vi "Do Action.vi"(8 "error in (no error)":errorcluster, 9 "Display Queue":refnum<queue>, 10 "tlc_User Event Reference.ctl":T1, 11 "Stop in":refnum<class "Stop.lvclass">) -> (0 "error out":errorcluster)   [LabVIEW 2010, in "Stop.lvclass"]
doc: "When the user clicks on the Stop button, this function will be called to halt execution of the cues that have been recorded in the Cue List."
uses:
  Stop.lvclass
  Controls/tlc_User Interface Command.ctl
  Controls/tlc_User Interface Data Type.ctl
  Controls/tlc_User Event Reference.ctl
  Play/Play.lvclass
  Stop.lvclass/Stop.ctl
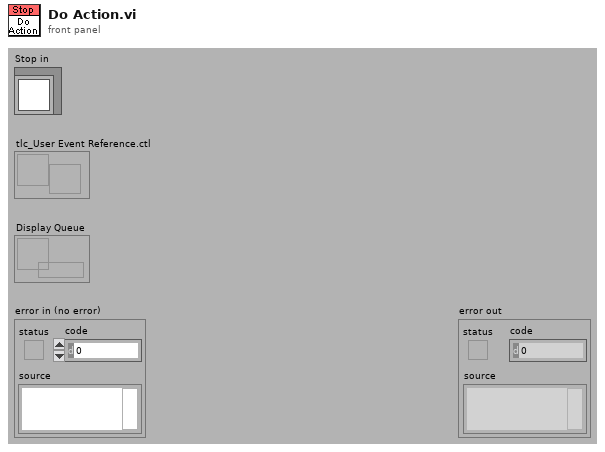
[diagram p1: front panel]
types:
  T1 = typedef "tlc_User Event Reference.ctl" = refnum<user-event>
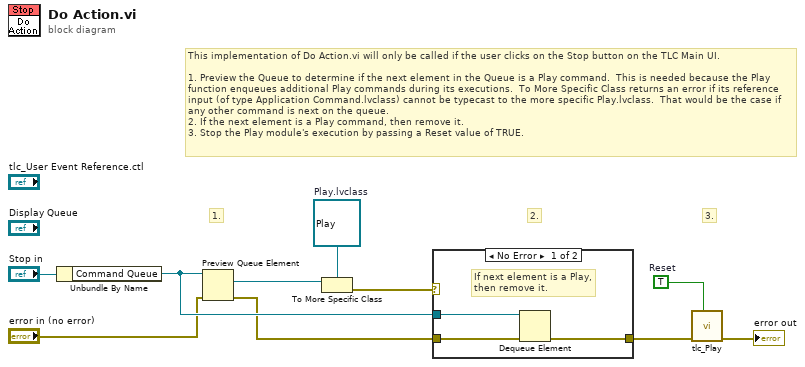
[diagram p0: block diagram]
diagram:
  w6 = refnum<class "Play.lvclass"> refnum  # Play.lvclass
  w10 = TRUE  # Reset
  # "3."
  # "2."
  # "1."
  # "This implementation of Do Action.vi will only be called if the user clicks on the Stop button on the TLC Main UI.  \n\n1. Preview the Queue to determine if the next element in the Queue is a Play command.  This is needed because the Play function enqueues additional Play commands during its executions.  To More Specific Class returns an error if its reference input (of type Application Command.lvclass) cannot be typecast to the more specific Play.lvclass.  That would be the case if any other command is next on the queue.\n2. If the next element is a Play command, then remove it.\n3. Stop the Play module's execution by passing a Reset value of TRUE."
  n1 = Unbundle By Name "Unbundle By Name"("Stop in") -> ("Command Queue"=w4:refnum<queue>)
  n2 = Preview Queue Element(queue=w4, error in (no error)="error in (no error)") -> (element=w7:refnum<class "Application Command.lvclass">, error out=w3:errorcluster)  [unwired: 1 in, 2 out]
  n3 = To More Specific Class(target class=w6, reference=w7) -> (error out=w5:errorcluster)  [unwired: 1 in, 1 out]
  n4 = case shown="No Error" w5 {
    tunnel: w4 -> [w13 _]
    tunnel: w3 -> [w12 w14]
    tunnel: [w11 w14] -> w1
    frame No Error {
      # "If next element is a Play,\nthen remove it."
      n5 = Dequeue Element(queue=w13, error in (no error)=w12) -> (error out=w11:errorcluster)  [unwired: 1 in, 3 out]
    }
    frame Error {
      # "This case executes if any command other than Play is next in the queue."
    }
  }
  n6 = call "tlc_Play.vi"("Reset"=w10, "error in (no error)"=w1) -> ("error out"=→"error out":errorcluster)  [unwired: 8 in, 1 out]
